vi "Teleop.vi"(10 "Match Info":T1={"Autonomous Elapsed Seconds"=0.0, "TeleOp Elapsed Seconds"=0.0, "Disabled Elapsed Seconds"=0.0, "Visited Autonomous"=FALSE, "Visited TeleOp"=FALSE, "Visited Disabled"=FALSE, "Autonomous Settings"={"Autonomous Style"=enum."Independent", "VI Refnum"=refnum}}, 11 "Call Context":T2) -> ()   [LabVIEW 2013]
doc: "This VI is called for each TeleOp packet received from the DS where the robot is not disabled. It is often used to read from the joysticks and update I/O or to update setpoints for timed control loops. It should complete and return within 20 milliseconds or it may miss DS packets."
uses:
  <vilib>/Rock Robotics/WPI/DriverStation/WPI_DriverStationDerivedRobotMode.ctl
  <vilib>/Rock Robotics/WPI/DriverStation/WPI_DriverStationMatch Info.ctl
  <vilib>/Rock Robotics/WPI/Solenoid/WPI_SolenoidValue.ctl
  Robot Global Data.vi
  <vilib>/Rock Robotics/WPI/Solenoid/Deprecated/WPI_SolenoidGetBool.vi
  <vilib>/Rock Robotics/WPI/Solenoid/WPI_SolenoidSetEnum.vi
  POT.vi
  <vilib>/Rock Robotics/WPI/Joystick/WPI_JoystickGetSetRefNum.vi
  <vilib>/Rock Robotics/WPI/RobotDrive/WPI_RobotDriveGetSetRefNum.vi
panel:
  out "POT 2":dbl
  out "POT":dbl
  out "Numeric 1":dbl(slide) scale=0.0..100.0
  out "Boolean 2":bool
  out "Boolean 1":bool
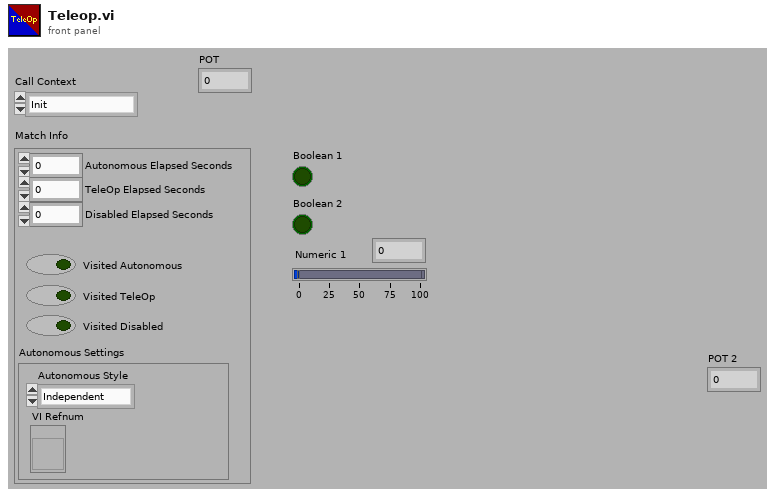
[diagram p1: front panel]
types:
  T1 = typedef "WPI_DriverStationMatch Info.ctl" = cluster{"Autonomous Elapsed Seconds":dbl, "TeleOp Elapsed Seconds":dbl, "Disabled Elapsed Seconds":dbl, "Visited Autonomous":bool, "Visited TeleOp":bool, "Visited Disabled":bool, "Autonomous Settings":cluster{"Autonomous Style":enum16{"Iterative", "Independent"}, "VI Refnum":refnum<vi>}}
  T2 = typedef "WPI_DriverStationDerivedRobotMode.ctl" = enum16{"Init", "Execute", "Stop"}
  T3 = typedef "WPI_JoystickDevRef.ctl" = cluster{"Device":T4}
  T4 = typedef "WPI_JoystickDeviceEnum.ctl" = enum16{"USB 1", "USB 2", "USB 3", "USB 4", "Kinect 1", "Kinect 2"}
  T5 = typedef "WPI_JoystickButtonState.ctl" = cluster{"Button 1":bool, "Button 2":bool, "Button 3":bool, "Button 4":bool, "Button 5":bool, "Button 6":bool, "Button 7":bool, "Button 8":bool, "Button 9":bool, "Button 10":bool, "Button 11":bool, "Button 12":bool}
  T6 = typedef "WPI_SolenoidDevRef.ctl" = cluster{"DevStatus":errorcluster, "Solenoid Module":T7, "Forward Solenoid Channel":T8, "Reverse Solenoid Channel":T8}
  T7 = typedef "FPGA_TypedefSolenoidModule.ctl" = enum16{"Solenoid Module 1", "Solenoid Module 2"}
  T8 = typedef "WPI_SolenoidChannel.ctl" = enum8{"Solenoid 1", "Solenoid 2", "Solenoid 3", "Solenoid 4", "Solenoid 5", "Solenoid 6", "Solenoid 7", "Solenoid 8", "Invalid"}
  T9 = typedef "WPI_SolenoidValue.ctl" = enum16{"Off", "On", "Forward", "Reverse"}
  T10 = typedef "WPI_MotorControlDeviceRef.ctl" = cluster{"DeviceStatus":errorcluster, "Type":enum16{"PWM", "CAN"}, "PWM":cluster{"Digital Module":T11, "PWM Channel":T12, "DeadBand":T13}, "CAN":cluster{"Device Number":u8, "Control Mode":T14, "Semaphore":T15, "Max Vout":dbl}, "Invert":bool, "TransformRef":T16, "InvTransformRef":T16}
  T11 = typedef "FPGA_TypedefDigitalModule.ctl" = enum16{"Digital Module 1", "Digital Module 2"}
  T12 = typedef "FPGA_DIOPWMChannel.ctl" = enum8{"PWM 1", "PWM 2", "PWM 3", "PWM 4", "PWM 5", "PWM 6", "PWM 7", "PWM 8", "PWM 9", "PWM 10", "Invalid"}
  T13 = typedef "WPI_PWMDeadband.ctl" = cluster{"Name":string, "maxPositivePwm":i32, "minPositivePwm":i32, "centerPwm":i32, "maxNegativePwm":i32, "minNegativePwm":i32, "angularRange":u16}
  T14 = typedef "WPI_CANJaguar_ControlMode.ctl" = enum8{"Percent VBus", "Current", "Speed", "Position", "Voltage"}
  T15 = typedef "Semaphore RefNum" = refnum<k1>
  T16 = typedef "WPI_PWMTransform_ConPane.ctl" = refnum<vi>
  T17 = typedef "WPI_RobotDriveDevRef.ctl" = cluster{"DevStatus":errorcluster, "Motors[]":T10[], "Square Inputs":bool, "Max Output":dbl, "Isochronous":bool}
  T18 = cluster{"axis 1 (x)":dbl, "axis 2 (y)":dbl, "axis 3 (throttle)":dbl, "axis 4":dbl, "axis 5":dbl, "axis 6":dbl}
  T19 = typedef "WPI_RelayDevRef.ctl" = cluster{"DevStatus":errorcluster, "Relay Channel":T20, "Digital Module":T11, "Relay Direction":T21}
  T20 = typedef "FPGA_DIORelayChannel.ctl" = enum8{"Relay 1", "Relay 2", "Relay 3", "Relay 4", "Relay 5", "Relay 6", "Relay 7", "Relay 8", "Invalid"}
  T21 = typedef "WPI_RelayDirection.ctl" = enum16{"Both directions", "Forward only", "Reverse only"}
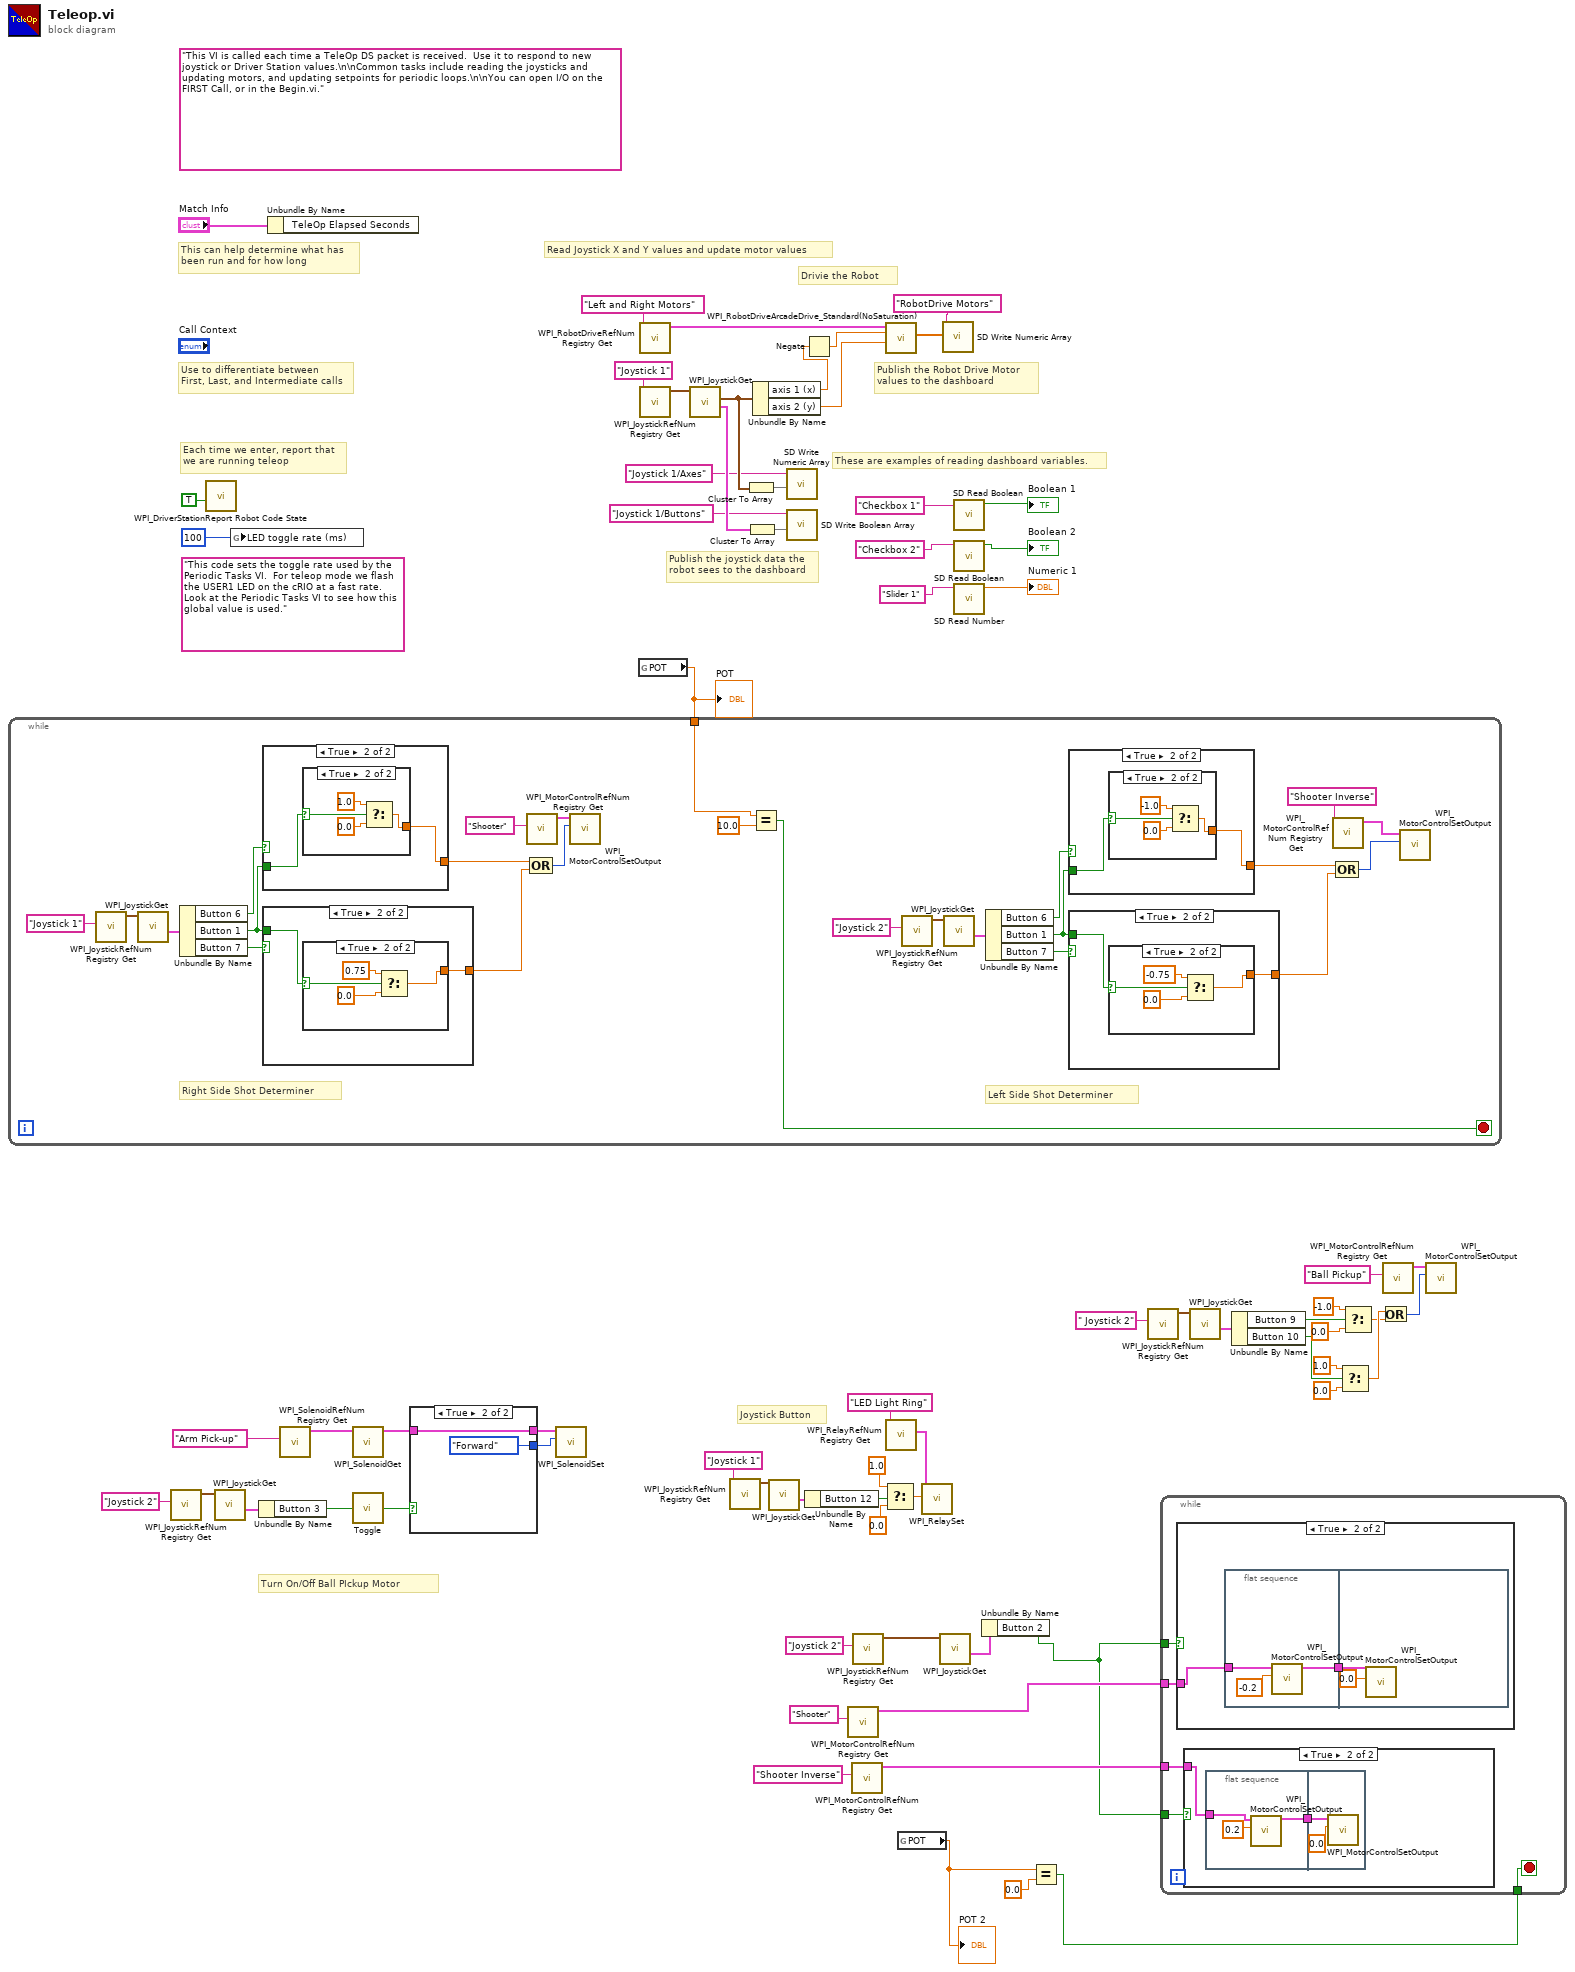
[diagram p0: block diagram]
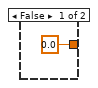
[diagram p2: hidden frame]
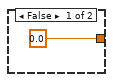
[diagram p3: hidden frame]
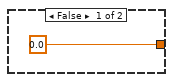
[diagram p4: hidden frame]
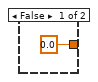
[diagram p5: hidden frame]
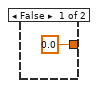
[diagram p6: hidden frame]
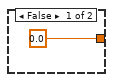
[diagram p7: hidden frame]
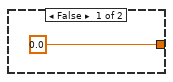
[diagram p8: hidden frame]
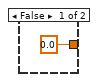
[diagram p9: hidden frame]
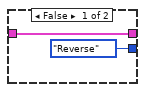
[diagram p12: hidden frame]
diagram:
  (unwired) "This code sets the toggle rate used by the Periodic Tasks VI.  For teleop mode we flash the USER1 LED on the cRIO at a fast rate.  Look at the Periodic Tasks VI to see how this global value is used."
  (unwired) "This VI is called each time a TeleOp DS packet is received.  Use it to respond to new joystick or Driver Station values.\n\nCommon tasks include reading the joysticks and updating motors, and updating setpoints for periodic loops.\n\nYou can open I/O on the FIRST Call, or in the Begin.vi."
  # "Turn On/Off Ball PIckup Motor"
  # "Joystick Button"
  # "Drivie the Robot"
  # "These are examples of reading dashboard variables."
  # "Publish the Robot Drive Motor\nvalues to the dashboard"
  # "Publish the joystick data the\nrobot sees to the dashboard"
  # "Each time we enter, report that\nwe are running teleop"
  # "Use to differentiate between\nFirst, Last, and Intermediate calls"
  # "This can help determine what has\nbeen run and for how long"
  # "Read Joystick X and Y values and update motor values"
  n1 = call <vilib>:"WPI_JoystickRefNum Registry Get.vi"("refnum name"="Joystick 2") -> ("JoystickDevRef"=w34:T3)  [unwired: 9 in, 1 out]
  n2 = call <vilib>:"WPI_DriverStationReport Robot Code State.vi"("TeleOp"=TRUE ("Autonomous")) -> ()  [unwired: 10 in, 1 out]
  n3 = call <vilib>:"WPI_JoystickGet.vi"("JoystickDevRef"=w34) -> ("Buttons"=w33:T5)  [unwired: 4 in, 2 out]
  n4 = global write "Robot Global Data.vi" "LED toggle rate (ms)"(u32 100 ("LED ms toggle rate")) -> ()
  n5 = Unbundle By Name(w33) -> ("Button 3"=w30:bool)
  n6 = Unbundle By Name("Match Info") -> ()  [unwired: 1 out]
  n7 = call <vilib>:"WPI_SolenoidRefNum Registry Get.vi"("refnum name"="Arm Pick-up") -> ("SolenoidDevRef"=w17:T6)  [unwired: 9 in, 1 out]
  n8 = call-poly <vilib>:"WPI_SolenoidGet.vi"("SolenoidDevRef"=w17) -> ("SolenoidDevRef"=w15:T6)  [unwired: 8 in, 2 out]
  n9 = call "Toggle.vi"("Input"=w30) -> ("Toggled Output"=w16:bool)
  n10 = case shown="True" w16 {
    tunnel: w15 -> [w71 w73]
    tunnel: [w71 w73] -> w14
    tunnel: [WPI_SolenoidValue."Reverse" ("Value") WPI_SolenoidValue."Forward" ("Value")] -> w13
    frame False {
    }
    frame True {
    }
  }
  n11 = call-poly <vilib>:"WPI_SolenoidSet.vi"("Value"=w13, "SolenoidDevRef"=w14) -> ()  [unwired: 8 in, 2 out]
  n12 = global read "POT.vi" "POT"() -> (w1:dbl)
  "POT" <- w1
  n13 = while {
    tunnel: w1 -> [w75]
    stop <- w74 stop-if-true
    # "Left Side Shot Determiner"
    # "Right Side Shot Determiner"
    n14 = call <vilib>:"WPI_JoystickRefNum Registry Get.vi"("refnum name"="Joystick 1") -> ("JoystickDevRef"=w97:T3)  [unwired: 9 in, 1 out]
    n15 = call <vilib>:"WPI_JoystickGet.vi"("JoystickDevRef"=w97) -> ("Buttons"=w96:T5)  [unwired: 4 in, 2 out]
    n16 = Unbundle By Name(w96) -> ("Button 6"=w95:bool, "Button 1"=w93:bool, "Button 7"=w94:bool)
    n17 = case shown="True" w95 {
      tunnel: w93 -> [_ w125]
      tunnel: [0.0 ("f") w124] -> w92
      frame False {
      }
      frame True {
        n18 = case shown="True" w125 {
          selector: w125 -> [_ w128]
          tunnel: [0.0 ("f") w127] -> w124
          frame False {
          }
          frame True {
            n19 = Select(t=1.0, s=w128, f=0.0) -> (s? t:f=w127:dbl)
          }
        }
      }
    }
    n20 = case shown="True" w94 {
      tunnel: w93 -> [_ w117]
      tunnel: [0.0 ("f") w116] -> w91
      frame False {
      }
      frame True {
        n21 = case shown="True" w117 {
          selector: w117 -> [_ w120]
          tunnel: [0.0 ("f") w119] -> w116
          frame False {
          }
          frame True {
            n22 = Select(t=0.75, s=w120, f=0.0) -> (s? t:f=w119:dbl)
          }
        }
      }
    }
    n23 = call <vilib>:"WPI_MotorControlRefNum Registry Get.vi"("refnum name"="Shooter") -> ("MotorControlDevRef"=w88:T10)  [unwired: 9 in, 1 out]
    n24 = Compound Arithmetic op=OR(w92, w91) -> (w90:i32)
    n25 = call <vilib>:"WPI_MotorControlSetOutput.vi"("Output"=w90, "MotorControlDevRef"=w88) -> ()  [unwired: 7 in, 3 out]
    n26 = Equal?(x=w75, y=10.0) -> (x = y?=w74:bool)
    n27 = call <vilib>:"WPI_JoystickRefNum Registry Get.vi"("refnum name"="Joystick 2") -> ("JoystickDevRef"=w78:T3)  [unwired: 9 in, 1 out]
    n28 = call <vilib>:"WPI_JoystickGet.vi"("JoystickDevRef"=w78) -> ("Buttons"=w79:T5)  [unwired: 4 in, 2 out]
    n29 = Unbundle By Name(w79) -> ("Button 6"=w80:bool, "Button 1"=w82:bool, "Button 7"=w81:bool)
    n30 = case shown="True" w80 {
      tunnel: w82 -> [_ w109]
      tunnel: [0.0 ("f") w108] -> w83
      frame False {
      }
      frame True {
        n31 = case shown="True" w109 {
          selector: w109 -> [_ w112]
          tunnel: [0.0 ("f") w111] -> w108
          frame False {
          }
          frame True {
            n32 = Select(t=-1.0, s=w112, f=0.0) -> (s? t:f=w111:dbl)
          }
        }
      }
    }
    n33 = case shown="True" w81 {
      tunnel: w82 -> [_ w101]
      tunnel: [0.0 ("f") w100] -> w84
      frame False {
      }
      frame True {
        n34 = case shown="True" w101 {
          selector: w101 -> [_ w104]
          tunnel: [0.0 ("f") w103] -> w100
          frame False {
          }
          frame True {
            n35 = Select(t=-0.75, s=w104, f=0.0) -> (s? t:f=w103:dbl)
          }
        }
      }
    }
    n36 = call <vilib>:"WPI_MotorControlRefNum Registry Get.vi"("refnum name"="Shooter Inverse") -> ("MotorControlDevRef"=w87:T10)  [unwired: 9 in, 1 out]
    n37 = Compound Arithmetic op=OR(w83, w84) -> (w85:i32)
    n38 = call <vilib>:"WPI_MotorControlSetOutput.vi"("Output"=w85, "MotorControlDevRef"=w87) -> ()  [unwired: 7 in, 3 out]
  }
  n39 = call <vilib>:"WPI_RobotDriveRefNum Registry Get.vi"("refnum name"="Left and Right Motors") -> ("RobotDriveDevRef"=w67:T17)  [unwired: 1 in, 9 out]
  n40 = call <vilib>:"WPI_JoystickRefNum Registry Get.vi"("refnum name"="Joystick 1") -> ("JoystickDevRef"=w64:T3)  [unwired: 1 in, 9 out]
  n41 = call <vilib>:"WPI_JoystickGet.vi"("JoystickDevRef"=w64) -> ("Buttons"=w61:T5, "Axes"=w58:T18)  [unwired: 1 in, 4 out]
  n42 = call <vilib>:"WPI_JoystickRefNum Registry Get.vi"("refnum name"="Joystick 1") -> ("JoystickDevRef"=w43:T3)  [unwired: 9 in, 1 out]
  n43 = Cluster To Array(cluster=w58) -> (array=w57:dbl[])
  n44 = Cluster To Array(cluster=w61) -> (array=w60:bool[])
  n45 = Unbundle By Name(w58) -> ("axis 1 (x)"=w32:dbl, "axis 2 (y)"=w66:dbl)
  n46 = call <vilib>:"WPI_JoystickGet.vi"("JoystickDevRef"=w43) -> ("Buttons"=w42:T5)  [unwired: 4 in, 2 out]
  n47 = call <vilib>:"SD Write Numeric Array.vi"("Numeric Array"=w57, "Name"="Joystick 1/Axes") -> ()  [unwired: 8 in, 2 out]
  n48 = call <vilib>:"SD Write Boolean Array.vi"("Boolean Array"=w60, "Name"="Joystick 1/Buttons") -> ()  [unwired: 8 in, 2 out]
  n49 = Negate(x=w32) -> (-x=w31:dbl)
  n50 = Unbundle By Name(w42) -> ("Button 12"=w41:bool)
  n51 = call <vilib>:"WPI_MotorControlRefNum Registry Get.vi"("refnum name"="Shooter") -> ("MotorControlDevRef"=w8:T10)  [unwired: 9 in, 1 out]
  n52 = call <vilib>:"WPI_MotorControlRefNum Registry Get.vi"("refnum name"="Shooter Inverse") -> ("MotorControlDevRef"=w4:T10)  [unwired: 9 in, 1 out]
  n53 = call <vilib>:"WPI_JoystickRefNum Registry Get.vi"("refnum name"="Joystick 2") -> ("JoystickDevRef"=w9:T3)  [unwired: 9 in, 1 out]
  n54 = Select(t=1.0, s=w41, f=0.0) -> (s? t:f=w40:dbl)
  n55 = call <vilib>:"WPI_RobotDriveArcadeDrive_Standard(NoSaturation).vi"("Y axis value"=w66, "X axis value"=w31, "RobotDriveDevRef"=w67) -> ("Motor Values"=w54:dbl[])  [unwired: 1 in, 7 out]
  n56 = call <vilib>:"WPI_RelayRefNum Registry Get.vi"("refnum name"="LED Light Ring") -> ("RelayDevRef"=w47:T19)  [unwired: 9 in, 1 out]
  n57 = global read "POT.vi" "POT"() -> (w6:dbl)
  "POT 2" <- w6
  n58 = call <vilib>:"WPI_RelaySet.vi"("RelayValue"=w40, "RelayDevRef"=w47) -> ()  [unwired: 8 in, 2 out]
  n59 = call <vilib>:"WPI_JoystickGet.vi"("JoystickDevRef"=w9) -> ("Buttons"=w7:T5)  [unwired: 4 in, 2 out]
  n60 = call <vilib>:"SD Write Numeric Array.vi"("Numeric Array"=w54, "Name"="RobotDrive Motors") -> ()  [unwired: 8 in, 2 out]
  n61 = call <vilib>:"SD Read Boolean.vi"("Name"="Checkbox 1" ("refnum name")) -> ("Boolean"=→"Boolean 1":bool)  [unwired: 8 in, 2 out]
  n62 = call <vilib>:"SD Read Boolean.vi"("Name"="Checkbox 2" ("refnum name")) -> ("Boolean"=→"Boolean 2":bool)  [unwired: 8 in, 2 out]
  n63 = call <vilib>:"SD Read Number.vi"("Name"="Slider 1" ("refnum name")) -> ("Numeric"=→"Numeric 1":dbl)  [unwired: 8 in, 2 out]
  n64 = Unbundle By Name(w7) -> ("Button 2"=w3:bool)
  n65 = Equal?(x=w6, y=0.0) -> (x = y?=w2:bool)
  n66 = call <vilib>:"WPI_JoystickRefNum Registry Get.vi"("refnum name"=" Joystick 2") -> ("JoystickDevRef"=w23:T3)  [unwired: 9 in, 1 out]
  n67 = while {
    tunnel: w8 -> [w135]
    tunnel: w3 -> [w134]
    tunnel: w4 -> [w133]
    tunnel: w3 -> [w132]
    tunnel: w2 -> [w131]
    stop <- w131 stop-if-true
    n68 = case shown="True" w134 {
      tunnel: w135 -> [_ w143]
      frame False {
      }
      frame True {
        n69 = flat-sequence {
          tunnel: [w146] -> w144
          tunnel: w143 -> [w145]
          tunnel: w144 -> [w149]
          frame #0 {
            n70 = call <vilib>:"WPI_MotorControlSetOutput.vi"("Output"=-0.2, "MotorControlDevRef"=w145) -> ("MotorControlDevRef"=w146:T10)  [unwired: 7 in, 2 out]
          }
          frame #1 {
            n71 = call <vilib>:"WPI_MotorControlSetOutput.vi"("Output"=0.0, "MotorControlDevRef"=w149) -> ()  [unwired: 7 in, 3 out]
          }
        }
      }
    }
    n72 = case shown="True" w132 {
      tunnel: w133 -> [_ w136]
      frame False {
      }
      frame True {
        n73 = flat-sequence {
          tunnel: [w139] -> w137
          tunnel: w136 -> [w138]
          tunnel: w137 -> [w141]
          frame #0 {
            n74 = call <vilib>:"WPI_MotorControlSetOutput.vi"("Output"=0.2, "MotorControlDevRef"=w138) -> ("MotorControlDevRef"=w139:T10)  [unwired: 7 in, 2 out]
          }
          frame #1 {
            n75 = call <vilib>:"WPI_MotorControlSetOutput.vi"("Output"=0.0, "MotorControlDevRef"=w141) -> ()  [unwired: 7 in, 3 out]
          }
        }
      }
    }
  }
  n76 = call <vilib>:"WPI_JoystickGet.vi"("JoystickDevRef"=w23) -> ("Buttons"=w24:T5)  [unwired: 4 in, 2 out]
  n77 = Unbundle By Name(w24) -> ("Button 9"=w25:bool, "Button 10"=w21:bool)
  n78 = Select(t=1.0, s=w21, f=0.0) -> (s? t:f=w20:dbl)
  n79 = Select(t=-1.0, s=w25, f=0.0) -> (s? t:f=w19:dbl)
  n80 = Or(x=w20, y=w19) -> (x .or. y?=w18:i32)
  n81 = call <vilib>:"WPI_MotorControlRefNum Registry Get.vi"("refnum name"="Ball Pickup") -> ("MotorControlDevRef"=w37:T10)  [unwired: 9 in, 1 out]
  n82 = call <vilib>:"WPI_MotorControlSetOutput.vi"("Output"=w18, "MotorControlDevRef"=w37) -> ()  [unwired: 7 in, 3 out]
